vi "Index Pulsing Interrupt - Reset On.vi"(11 "IRQ Number":u8) -> ()   [LabVIEW 2018]
panel:
  out "Stop?":bool
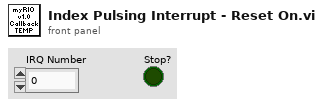
[diagram p1: front panel]
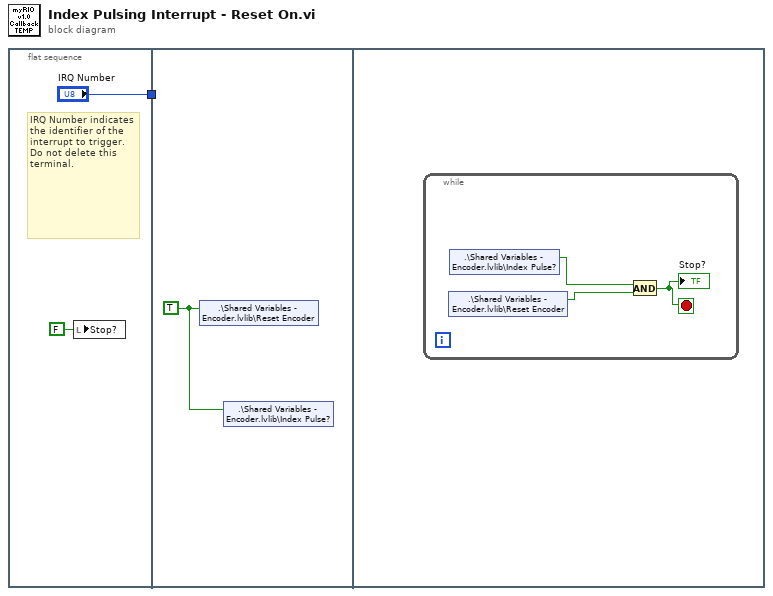
[diagram p0: block diagram]
diagram:
  n1 = flat-sequence {
    tunnel: ["IRQ Number"] -> w1
    tunnel: w1 -> [_]
    frame #0 {
      # "IRQ Number indicates the identifier of the interrupt to trigger. Do not delete this terminal."
      n2 = local write "Stop?"(FALSE ("Stop?")) -> ()
    }
    frame #1 {
      w4 = TRUE ("Reset Encoder")
      n3 = shared-variable ".\\Shared Variables - Encoder.lvlib\\Reset Encoder"(w4) -> ()  [unwired: 1 in, 1 out]
      n4 = shared-variable ".\\Shared Variables - Encoder.lvlib\\Index Pulse?"(w4) -> ()  [unwired: 1 in, 1 out]
    }
    frame #2 {
      n5 = while {
        stop <- w5 stop-if-true
        n6 = shared-variable ".\\Shared Variables - Encoder.lvlib\\Reset Encoder"() -> (w6:bool)  [unwired: 1 in, 1 out]
        n7 = shared-variable ".\\Shared Variables - Encoder.lvlib\\Index Pulse?"() -> (w7:bool)  [unwired: 1 in, 1 out]
        n8 = And(x=w7, y=w6) -> (x .and. y?=w5:bool)
        "Stop?" <- w5
      }
    }
  }
